vi "Persistent Switch Values.vi"(3 "Persistence Status In":string, 4 "Persistent Field In":dbl format="%.2f", 5 "Persistence In":bool, 6 "Read/Write":bool) -> (0 "Persistence Status Out":string, 1 "Persistence Out":bool, 2 "Persistent Field Out":dbl format="%.2f")   [LabVIEW 2025]
doc: "Author: Scott Hannahs <sth@magnet.fsu.edu>\n\nThis software is licensed for use under the “MIT License\"\nCopyright (c) 2025 Scott Hannahs, sth@sth@magnet.sthnet.net\n\nPermission is hereby granted, free of charge, to any person obtaining a copy of this software and associated documentation files (the \"Software\"), to deal in the Software without restriction, including without limitation the rights to use, copy, modify, merge, publish, distribute, sublicense, and/or sell copies of the Software, and to permit persons to whom the Software is furnished to do so, subject to the following conditions: The above copyright notice and this permission notice shall be included in all copies or substantial portions of the Software.\n\nTHE SOFTWARE IS PROVIDED \"AS IS\", WITHOUT WARRANTY OF ANY KIND, EXPRESS OR IMPLIED, INCLUDING BUT NOT LIMITED TO THE WARRANTIES OF MERCHANTABILITY, FITNESS FOR A PARTICULAR PURPOSE AND NONINFRINGEMENT. IN NO EVENT SHALL THE AUTHORS OR COPYRIGHT HOLDERS BE LIABLE FOR ANY CLAIM, DAMAGES OR OTHER LIABILITY, WHETHER IN AN ACTION OF CONTRACT, TORT OR OTHERWISE, ARISING FROM, OUT OF OR IN CONNECTION WITH THE SOFTWARE OR THE USE OR OTHER DEALINGS IN THE SOFTWARE."
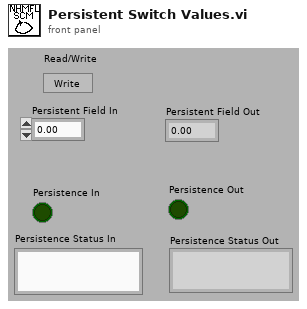
[diagram p1: front panel]
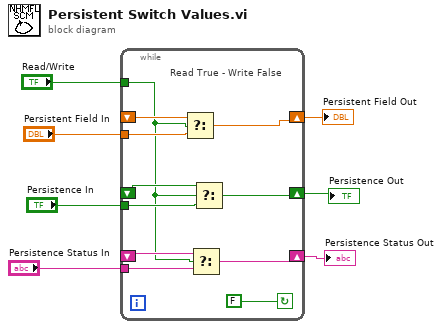
[diagram p0: block diagram]
diagram:
  n1 = while {
    shift-right: [w17] -> w4
    shift-left: _ -> [w16]
    shift-right: [w14] -> w3
    shift-left: _ -> [w15]
    tunnel: "Read/Write" -> [w8]
    tunnel: "Persistent Field In" -> [w18]
    tunnel: "Persistence In" -> [w13]
    shift-right: [w10] -> w1
    shift-left: _ -> [w9]
    tunnel: "Persistence Status In" -> [w11]
    stop <- FALSE continue-if-true
    # "Read True - Write False"
    n2 = Select(t=w16, s=w8, f=w18) -> (s? t:f=w17:dbl)
    n3 = Select(t=w9, s=w8, f=w11) -> (s? t:f=w10:string)
    n4 = Select(t=w15, s=w8, f=w13) -> (s? t:f=w14:bool)
  }
  "Persistence Out" <- w3
  "Persistent Field Out" <- w4
  "Persistence Status Out" <- w1
